vi "Faults.SetChannelFaultValue.vi"(9 "Fault Value to Set":dbl, 10 "Channel Name":string, 11 "GatewayIP":string) -> (0 "error out":errorcluster)   [LabVIEW 2013, in "MiscHelperVIs.lvlib"]
uses:
  MiscHelperVIs.lvlib
  <vilib>/NI Veristand/Execution/ChannelFaultManager/NI_VS ChannelFault ExecutionAPI.lvlib
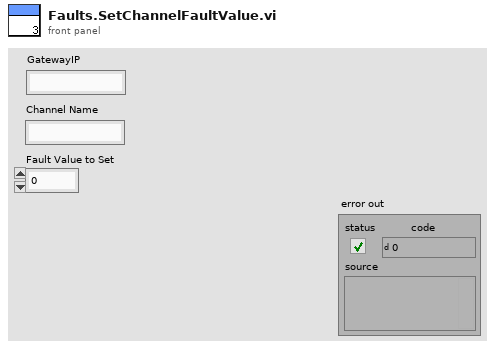
[diagram p1: front panel]
types:
  T1 = typedef "NI_VS ChannelFault ExecutionAPI.lvlib/ChannelFaultAPI.ctl" = refnum<k24>
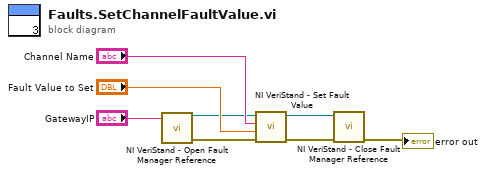
[diagram p0: block diagram]
diagram:
  n1 = call <vilib>:"NI VeriStand - Open Fault Manager Reference.vi"("Gateway IP Address (\"\": localhost)"="GatewayIP") -> ("error out"=w7:errorcluster, "ChannelFault"=w4:T1)  [unwired: 9 in]
  n2 = call <vilib>:"NI VeriStand - Set Fault Value.vi"("error in (no error)"=w7, "Fault Value"="Fault Value to Set", "Channel"="Channel Name", "ChannelFault in"=w4) -> ("error out"=w3:errorcluster, "ChannelFault out"=w2:T1)  [unwired: 6 in]
  n3 = call <vilib>:"NI VeriStand - Close Fault Manager Reference.vi"("error in (no error)"=w3, "ChannelFault"=w2) -> ("error out"=→"error out":errorcluster)  [unwired: 9 in]
